vi "AutonRamp.vi"(9 "Target":dbl, 10 "Start":dbl, 11 "Rate":dbl) -> (3 "Out":dbl)   [LabVIEW 2014]
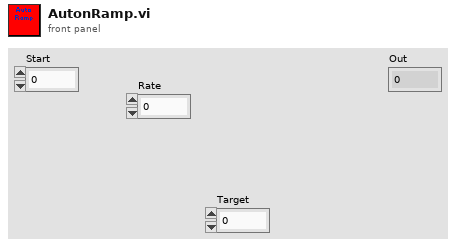
[diagram p1: front panel]
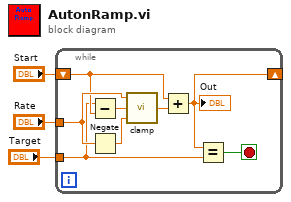
[diagram p0: block diagram]
diagram:
  n1 = while {
    shift-right: [w4] -> _
    shift-left: "Start" -> [w7]
    tunnel: "Target" -> [w6]
    tunnel: "Rate" -> [w9]
    stop <- w5 stop-if-true
    n2 = Subtract(x=w6, y=w7) -> (x-y=w11:dbl)
    n3 = Negate(x=w9) -> (-x=w10:dbl)
    n4 = call "clamp.vi"("Min"=w10, "Input"=w11, "Max"=w9) -> ("Output"=w8:dbl)
    n5 = Add(x=w7, y=w8) -> (x+y=w4:dbl)
    "Out" <- w4
    n6 = Equal?(x=w4, y=w6) -> (x = y?=w5:bool)
  }
